vi "GetCyclicFramesInformation.vi"(8 "error in (no error)":errorcluster, 11 "Device Ref in":T2 format="%.0x") -> (0 "error out":errorcluster, 1 "FR Signals":refnum<k21>[](array[refnum]), 2 "Channel Data Ref":T1[](array[typedef]) format="%.0x", 3 "Device Ref out":T2 format="%.0x")   [LabVIEW 2020, in "FlexRay Custom Device Engine.lvlib"]
uses:
  FlexRay Custom Device Engine.lvlib
  <vilib>/NI VeriStand/Custom Device API/Custom Device Item Ref.ctl
  <vilib>/NI VeriStand/Custom Device API/Data Reference.ctl
  <vilib>/NI VeriStand/Custom Device API/Data Access Type.ctl
  <vilib>/NI VeriStand/Custom Device API/Custom Device API.lvlib
  <vilib>/NI VeriStand/Custom Device Tools/Custom Device Utility Library/Custom Device Utility Library.lvlib
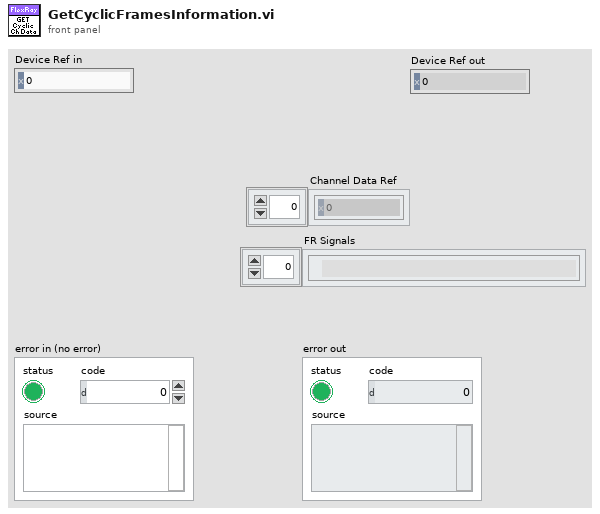
[diagram p1: front panel]
types:
  T1 = typedef "Custom Device API.lvlib/Data Reference.ctl" = i32
  T2 = typedef "Custom Device API.lvlib/Custom Device Item Ref.ctl" = u64
  T3 = typedef "Custom Device API.lvlib/Data Access Type.ctl" = enum16{"Read", "Write"}
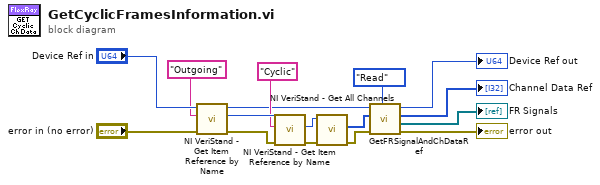
[diagram p0: block diagram]
diagram:
  n1 = call <vilib>:"NI VeriStand - Get Item Reference by Name.vi"("error in (no error)"="error in (no error)", "Item Name"="Outgoing" ("Section Name"), "Parent Ref in"="Device Ref in") -> ("error out"=w12:errorcluster, "Item Ref"=w16:T2, "Parent Ref out"=w7:T2)  [unwired: 5 in, 1 out]
  n2 = call <vilib>:"NI VeriStand - Get Item Reference by Name.vi"("error in (no error)"=w12, "Item Name"="Cyclic", "Parent Ref in"=w16) -> ("error out"=w11:errorcluster, "Item Ref"=w14:T2)  [unwired: 5 in, 2 out]
  n3 = call <vilib>:"NI VeriStand - Get All Channels.vi"("error in"=w11, "Section Ref in"=w14) -> ("error out"=w5:errorcluster, "Channel Refs"=w4:T2[])  [unwired: 6 in, 2 out]
  n4 = call "GetFRSignalAndChDataRef.vi"("Access"=Data_Access_Type."Read", "error in (no error)"=w5, "Channel Refs"=w4, "Device Ref in"=w7) -> ("error out"=→"error out":errorcluster, "FR Signals"=→"FR Signals":refnum<k21>[], "Channel Data Ref"=→"Channel Data Ref":T1[], "Device Ref out"=→"Device Ref out":T2)  [unwired: 4 in]
